vi "lfield_get_frame_from_queue.vi"(8 "error in (no error)":errorcluster, 10 "timeout":i32=-1, 11 "lightfield_class in":refnum<class "lightfield_class.lvclass">) -> (0 "error out":errorcluster, 2 "image_data":T1, 3 "lightfield_class out":refnum<class "lightfield_class.lvclass">)   [LabVIEW 2015, in "lightfield_class.lvclass"]
uses:
  lightfield_class.lvclass
  lightfield_class.lvclass/lightfield_class.ctl
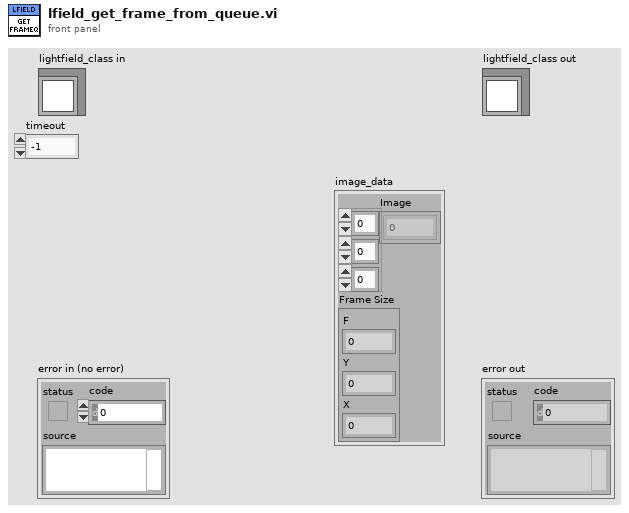
[diagram p1: front panel]
types:
  T1 = cluster{"Image":dbl[][][], "Frame Size":cluster{"F":i32, "Y":i32, "X":i32}}
  T2 = cluster{"Image":dbl[][][], "Frame Size":cluster{"F":i32, "Y":i32, "X":i32}}[]
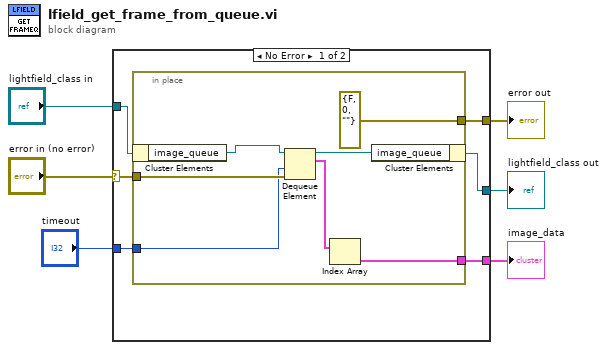
[diagram p0: block diagram]
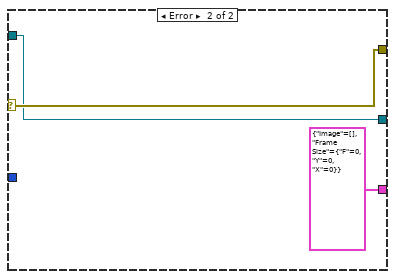
[diagram p2: hidden frame]
diagram:
  n1 = case shown="No Error" "error in (no error)" {
    selector: "error in (no error)" -> [w11 w22]
    tunnel: [w8 w22] -> w5
    tunnel: [w10 w21] -> w3
    tunnel: "lightfield_class in" -> [w12 w21]
    tunnel: [w9 T1 {"Image"=[], "Frame Size"={"F"=0, "Y"=0, "X"=0}} ("Cluster")] -> w2
    tunnel: "timeout" -> [w7 _]
    frame No Error {
      n2 = in-place {
        in-place-border: w11 -> [w17]
        in-place-border: [w15] -> w9
        in-place-border: [errorcluster {"status"=FALSE, "code"=0, "source"=""} ("error out")] -> w8
        in-place-border: w7 -> [w13]
        n3 = in-place-cluster #1(w12) -> ("image_queue"=w19:refnum<queue>)
        n4 = Dequeue Element(queue=w19, timeout in ms (-1)=w13, error in (no error)=w17) -> (queue out=w18:refnum<queue>, element=w16:T2)  [unwired: 2 out]
        n5 = Index Array(array=w16) -> (element=w15:T1)  [unwired: 1 in]
        n6 = in-place-cluster #1("image_queue"=w18) -> (w10:refnum<class "lightfield_class.lvclass">)
      }
    }
    frame Error {
    }
  }
  "error out" <- w5
  "lightfield_class out" <- w3
  "image_data" <- w2
